vi "Add Task Control Tree.vi"(8 "error in (no error)":errorcluster, 11 "Item Ref in":T1 format="%.0x") -> (0 "error out":errorcluster, 3 "Parent Ref out":T1 format="%.0x")   [LabVIEW 2020, in "Vires VTD System Explorer.lvlib"]
uses:
  Vires VTD System Explorer.lvlib
  <vilib>/NI VeriStand/Custom Device API/Custom Device Item Ref.ctl
  <vilib>/NI VeriStand/Custom Device API/Custom Device Channel.ctl
  <vilib>/NI VeriStand/Custom Device API/Custom Device Channel Type.ctl
  Shared/Constants.vi
  <vilib>/NI VeriStand/Custom Device API/Custom Device API.lvlib
  Shared/Vires VTD Shared.lvlib
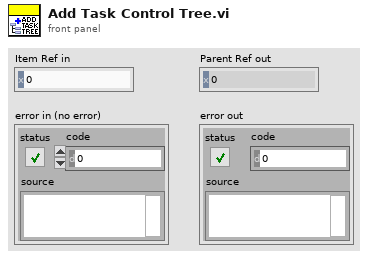
[diagram p1: front panel]
types:
  T1 = typedef "Custom Device API.lvlib/Custom Device Item Ref.ctl" = u64
  T2 = typedef "Custom Device API.lvlib/Custom Device Channel.ctl" = cluster{"Type":T3, "Units":string, "Default Value":dbl, "Faultable":bool, "Scalable":bool}
  T3 = typedef "Custom Device API.lvlib/Custom Device Channel Type.ctl" = enum16{"Input", "Output"}
  T4 = cluster{"Name":string, "Description":string, "Channel":T2}[]
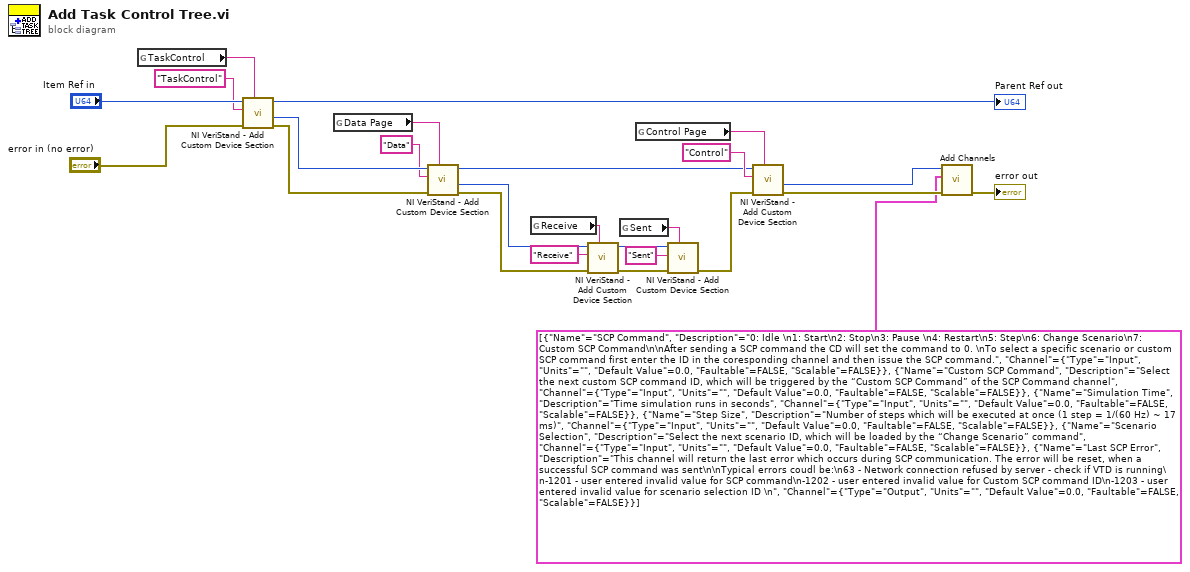
[diagram p0: block diagram]
diagram:
  n1 = global read "Constants.vi" "TaskControl"() -> (w18:string)
  n2 = call <vilib>:"NI VeriStand - Add Custom Device Section.vi"("GUID (Default Section)"=w18, "error in (no error)"="error in (no error)", "Section Name"="TaskControl", "Parent Ref in"="Item Ref in") -> ("error out"=w21:errorcluster, "Section Ptr"=w22:T1, "Parent Ref out"=→"Parent Ref out":T1)  [unwired: 4 in, 1 out]
  n3 = global read "Constants.vi" "Data Page"() -> (w15:string)
  n4 = call <vilib>:"NI VeriStand - Add Custom Device Section.vi"("GUID (Default Section)"=w15, "error in (no error)"=w21, "Section Name"="Data", "Parent Ref in"=w22) -> ("error out"=w5:errorcluster, "Section Ptr"=w17:T1, "Parent Ref out"=w12:T1)  [unwired: 4 in, 1 out]
  n5 = global read "Constants.vi" "Receive"() -> (w7:string)
  n6 = call <vilib>:"NI VeriStand - Add Custom Device Section.vi"("GUID (Default Section)"=w7, "error in (no error)"=w5, "Section Name"="Receive", "Parent Ref in"=w17) -> ("error out"=w8:errorcluster, "Parent Ref out"=w10:T1)  [unwired: 4 in, 2 out]
  n7 = global read "Constants.vi" "Sent"() -> (w6:string)
  n8 = global read "Constants.vi" "Control Page"() -> (w16:string)
  n9 = call <vilib>:"NI VeriStand - Add Custom Device Section.vi"("GUID (Default Section)"=w6, "error in (no error)"=w8, "Section Name"="Sent", "Parent Ref in"=w10) -> ("error out"=w25:errorcluster)  [unwired: 4 in, 3 out]
  n10 = call <vilib>:"NI VeriStand - Add Custom Device Section.vi"("GUID (Default Section)"=w16, "error in (no error)"=w25, "Section Name"="Control", "Parent Ref in"=w12) -> ("error out"=w3:errorcluster, "Section Ptr"=w4:T1)  [unwired: 4 in, 2 out]
  n11 = call "Add Channels.vi"("error in (no error)"=w3, "Channels Setup"=T4 [{"Name"="SCP Command", "Description"="0: Idle \n1: Start\n2: Stop\n3: Pause \n4: Restart\n5: Step\n6: Change Scenario\n7: Custom SCP Command\n\nAfter sending a SCP command the CD will set the command to 0. \nTo select a specific scenario or custom SCP command first enter the ID in the coresponding channel and then issue the SCP command.", "Channel"={"Type"=enum."Input", "Units"="", "Default Value"=0.0, "Faultable"=FALSE, "Scalable"=FALSE}}, {"Name"="Custom SCP Command", "Description"="Select the next custom SCP command ID, which will be triggered by the “Custom SCP Command” of the SCP Command channel", "Channel"={"Type"=enum."Input", "Units"="", "Default Value"=0.0, "Faultable"=FALSE, "Scalable"=FALSE}}, {"Name"="Simulation Time", "Description"="Time simulation runs in seconds", "Channel"={"Type"=enum."Input", "Units"="", "Default Value"=0.0, "Faultable"=FALSE, "Scalable"=FALSE}}, {"Name"="Step Size", "Description"="Number of steps which will be executed at once (1 step = 1/(60 Hz) ~ 17 ms)", "Channel"={"Type"=enum."Input", "Units"="", "Default Value"=0.0, "Faultable"=FALSE, "Scalable"=FALSE}}, {"Name"="Scenario Selection", "Description"="Select the next scenario ID, which will be loaded by the “Change Scenario” command", "Channel"={"Type"=enum."Input", "Units"="", "Default Value"=0.0, "Faultable"=FALSE, "Scalable"=FALSE}}, {"Name"="Last SCP Error", "Description"="This channel will return the last error which occurs during SCP communication. The error will be reset, when a successful SCP command was sent\n\nTypical errors coudl be:\n63 - Network connection refused by server - check if VTD is running\n-1201 - user entered invalid value for SCP command\n-1202 - user entered invalid value for Custom SCP command ID\n-1203 - user entered invalid value for scenario selection ID \n", "Channel"={"Type"=enum."Output", "Units"="", "Default Value"=0.0, "Faultable"=FALSE, "Scalable"=FALSE}}], "Section Ptr In"=w4) -> ("error out"=→"error out":errorcluster)  [unwired: 7 in, 1 out]
